vi "Dequeue Message.vi"(8 "error in (no error)":errorcluster, 11 "Message Queue":refnum<queue>) -> (0 "error out":errorcluster, 1 "Message Data":variant, 2 "Message":string, 3 "dup Message Queue":refnum<queue>)   [LabVIEW 2018, in "BMark_Message Queue.lvlib"]
doc: "This VI pulls messages off the Message Queue. It has special error handling to account for an error occurring on the last iteration of the Message Handling Loop.\n\nNo Error - normal Dequeue Element operation.\nError - check if it is an error code we wish to ignore. If so, clear the error and perform a normal Dequeue Element. If not, output the error, and put an 'Exit' message on the Message Queue."
uses:
  <resource>/dialog/BookmarkManager/managers/Default/support/Message Queue/BMark_Message Queue.lvlib
  <resource>/dialog/BookmarkManager/managers/Default/support/Message Queue/Message Cluster.ctl
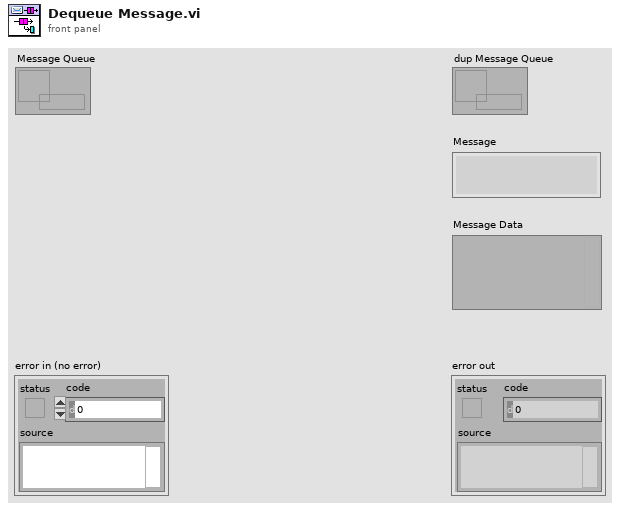
[diagram p1: front panel]
types:
  T1 = typedef "BMark_Message Queue.lvlib/Message Cluster.ctl" = cluster{"Message":string, "Message Data":variant}
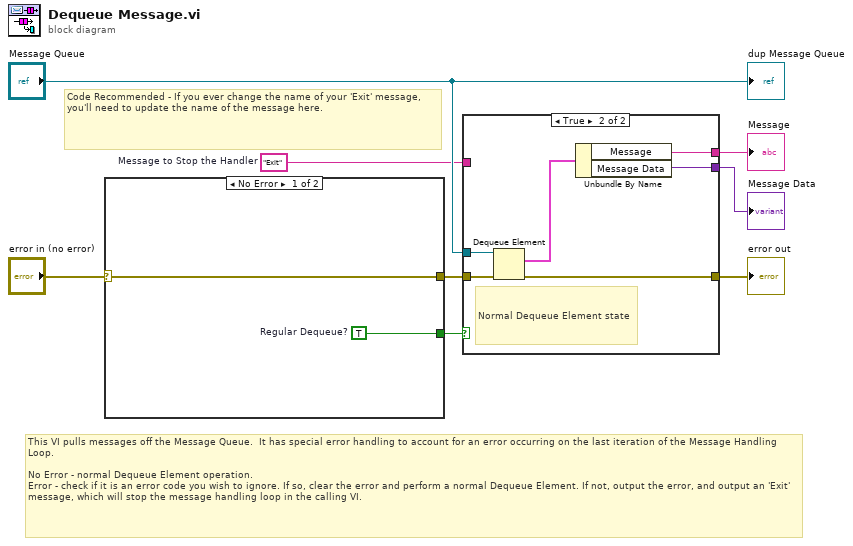
[diagram p0: block diagram]
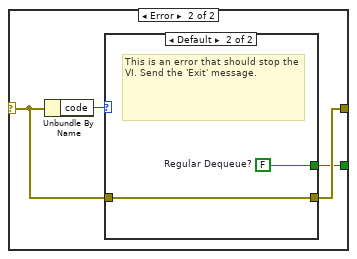
[diagram p3: hidden frame]
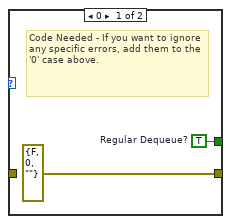
[diagram p4: hidden frame]
diagram:
  w1 = "Exit"  # Message to Stop the Handler
  # "Code Recommended - If you ever change the name of your 'Exit' message, you'll need to update the name of the message here."
  # "This VI pulls messages off the Message Queue.  It has special error handling to account for an error occurring on the last iteration of the Message Handling Loop.\n\nNo Error - normal Dequeue Element operation.\nError - check if it is an error code you wish to ignore. If so, clear the error and perform a normal Dequeue Element. If not, output the error, and output an 'Exit' message, which will stop the message handling loop in the calling VI."
  n1 = case shown="No Error" "error in (no error)" {
    selector: "error in (no error)" -> [w10 w13]
    tunnel: [w10 w12] -> w6
    tunnel: [w9 w11] -> w5
    frame No Error {
      w9 = TRUE  # Regular Dequeue?
    }
    frame Error {
      n2 = Unbundle By Name(w13) -> ("code"=w14:i32)
      n3 = case shown="Default" w14 {
        tunnel: [errorcluster {"status"=FALSE, "code"=0, "source"=""} ("error constant") w18] -> w12
        tunnel: w13 -> [_ w18]
        tunnel: [w16 w17] -> w11
        frame 0 {
          w16 = TRUE  # Regular Dequeue?
          # "Code Needed - If you want to ignore any specific errors, add them to the '0' case above."
        }
        frame Default {
          w17 = FALSE  # Regular Dequeue?
          # "This is an error that should stop the VI. Send the 'Exit' message."
        }
      }
    }
  }
  n4 = case shown="True" w5 {
    tunnel: [w20 w26] -> w7
    tunnel: w6 -> [w20 w25]
    tunnel: "Message Queue" -> [_ w24]
    tunnel: [w19 w22] -> w3
    tunnel: [_ w21] -> w2
    tunnel: w1 -> [w19 _]
    frame False {
    }
    frame True {
      # "Normal Dequeue Element state"
      n5 = Dequeue Element(queue=w24, error in (no error)=w25) -> (element=w23:T1, error out=w26:errorcluster)  [unwired: 1 in, 2 out]
      n6 = Unbundle By Name(w23) -> ("Message"=w22:string, "Message Data"=w21:variant)
    }
  }
  "error out" <- w7
  "Message" <- w3
  "Message Data" <- w2
  "dup Message Queue" <- "Message Queue"
